vi "dlw_Work Planer.vi"(6 "Worker Alias":string="Work Planer", 7 "Caller in":refnum<class "Worker.lvclass">, 8 "error in":errorcluster, 10 "Initialization Data":T1={"Response Cases"={"Timeout"=""}, "Time Precission (100ms)"=100, "Continius? (F)"=FALSE, "Data"=variant, "Auxiliary"=variant, "Priority (Normal)"=enum."Normal", "Timeout (1000ms)"=1000, "Debugger MSG? (T)"=TRUE}, 11 "Work Planer in":refnum<class "Work Planer.lvclass">) -> (0 "error out":errorcluster, 3 "Work Planer out":refnum<class "Work Planer.lvclass">, 5 "dup Caller out":refnum<class "Worker.lvclass">)   [LabVIEW 2018, in "Work Planer.lvclass"]
doc: "This VI dynamically loads the Worker that owns this VI as a subWorker into <b>Caller</b>, and returns the Worker's object containing the Worker's Public Properties. Initialization data that is to be received by this Worker's <Initialize> MHL case can be wired to <b>Initialization Data</b>. The dynamically loaded Worker requires an alias ( <b>Worker Alias</b> ) which must be unique to the Worker it is called from. If a currently loaded subWorker exists with the same Alias, an error will be returned.\n\n<b>Note:</b> This VI can only be used from <b>within</b> a Worker's MHL. To load this Worker from an external LabVIEW application or from TestStand, please use an Asynchronous Launcher VI.\n---"
uses:
  Work Planer.lvclass
  C:/Program Files (x86)/National Instruments/LabVIEW 2018/vi.lib/addons/_Workers/Library/Classes/Worker/Worker.lvclass
  <vilib>/addons/_Workers/Library/Classes/Worker/Worker.lvclass
  Initialization Data.ctl
  Response Cases.ctl
  <vilib>/addons/_Workers/Library/Case Label.ctl
  <vilib>/addons/_Workers/Library/Classes/Message/Priority (ALL).ctl
  <vilib>/addons/_Workers/Library/Workers.lvlib
  <vilib>/addons/_Workers/Library/Classes/Message/Message.lvclass
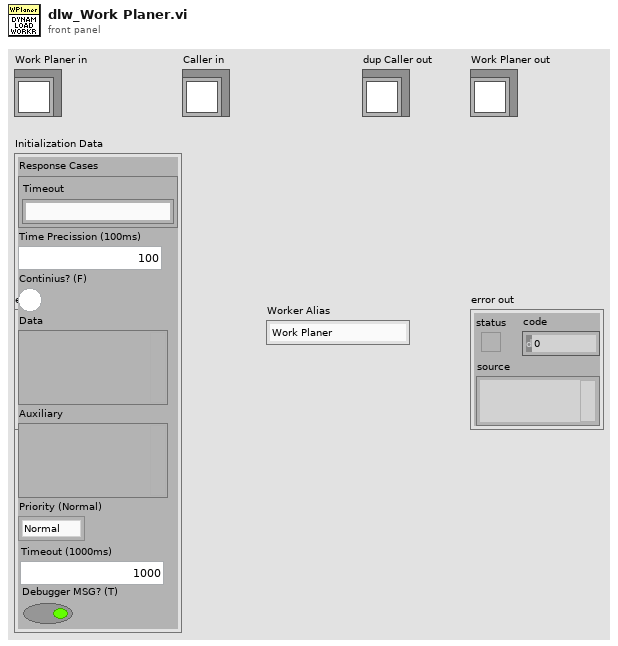
[diagram p1: front panel]
types:
  T1 = typedef "Work Planer.lvclass/Initialization Data.ctl" = cluster{"Response Cases":T2, "Time Precission (100ms)":u32, "Continius? (F)":bool, "Data":variant, "Auxiliary":variant, "Priority (Normal)":T4, "Timeout (1000ms)":u32, "Debugger MSG? (T)":bool}
  T2 = typedef "Work Planer.lvclass/Response Cases.ctl" = cluster{"Timeout":T3}
  T3 = typedef "Workers.lvlib/Case Label.ctl" = string
  T4 = typedef "Workers.lvlib/Message.lvclass/Priority (ALL).ctl" = enum16{"Low", "Normal", "High", "Critical"}
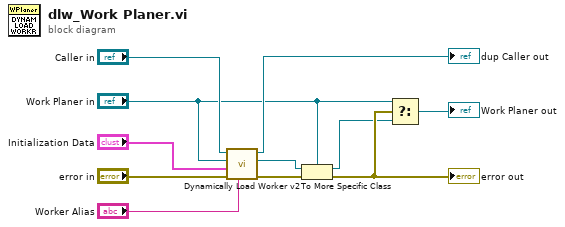
[diagram p0: block diagram]
diagram:
  n1 = call <vilib>:"Dynamically Load Worker v2.vi"("Worker Alias"="Worker Alias", "error in"="error in", "Initialization Data"="Initialization Data", "Worker to Dynamically Load"="Work Planer in", "Worker"="Caller in") -> ("error out"=w10:errorcluster, "Dynamically Loaded Worker out"=w5:refnum<class "Worker.lvclass">, "dup Worker out"=→"dup Caller out":refnum<class "Worker.lvclass">)  [unwired: 4 in]
  n2 = To More Specific Class(target class="Work Planer in", reference=w5, error in=w10) -> (specific class reference=w2:refnum<class "Work Planer.lvclass">, error out=w4:errorcluster)
  "error out" <- w4
  n3 = Select(t="Work Planer in", s=w4, f=w2) -> (s? t:f=→"Work Planer out":refnum<class "Work Planer.lvclass">)
